vi "Daemon_JETAbout.vi"(6 "Dialog Name":string, 10 "Dialog Parameters":string) -> ()   [LabVIEW 2019]
doc: "JSMA Module Template - Top Level UI 0.2.0.4\nRob Humfeld - Jet Engineering\nCopyright (c) 2019, Jet Engineering"
uses:
  Daemon_JETAbout - Status STYP.ctl
  <userlib>/Jet Labs/JET Panel/JETPanel_Behavior_STYP.ctl
  <userlib>/Jet Engineering/JET_QSM/Code/Private/JET_QSM - Add State [String API].vi
  <vilib>/Utility/error.llb/Trim Whitespace.vi
  <vilib>/Utility/error.llb/Error Cluster From Error Code.vi
  <userlib>/Jet Labs/JET Panel/JETPanel.lvclass
panel:
  in  "exit?":bool
  out "Prompt":string
  out "winSizer 2":string="W"
  out "winSizer 1":string="W"
  out "Recent states before Error (with tick counts) 2":string
  in  "Status":T1
  out "error out":errorcluster
  # "1241 Park Place NE, Ste E, Cedar Rapids, IA 52402\n319.294.6106        http://www.jetinc.net"
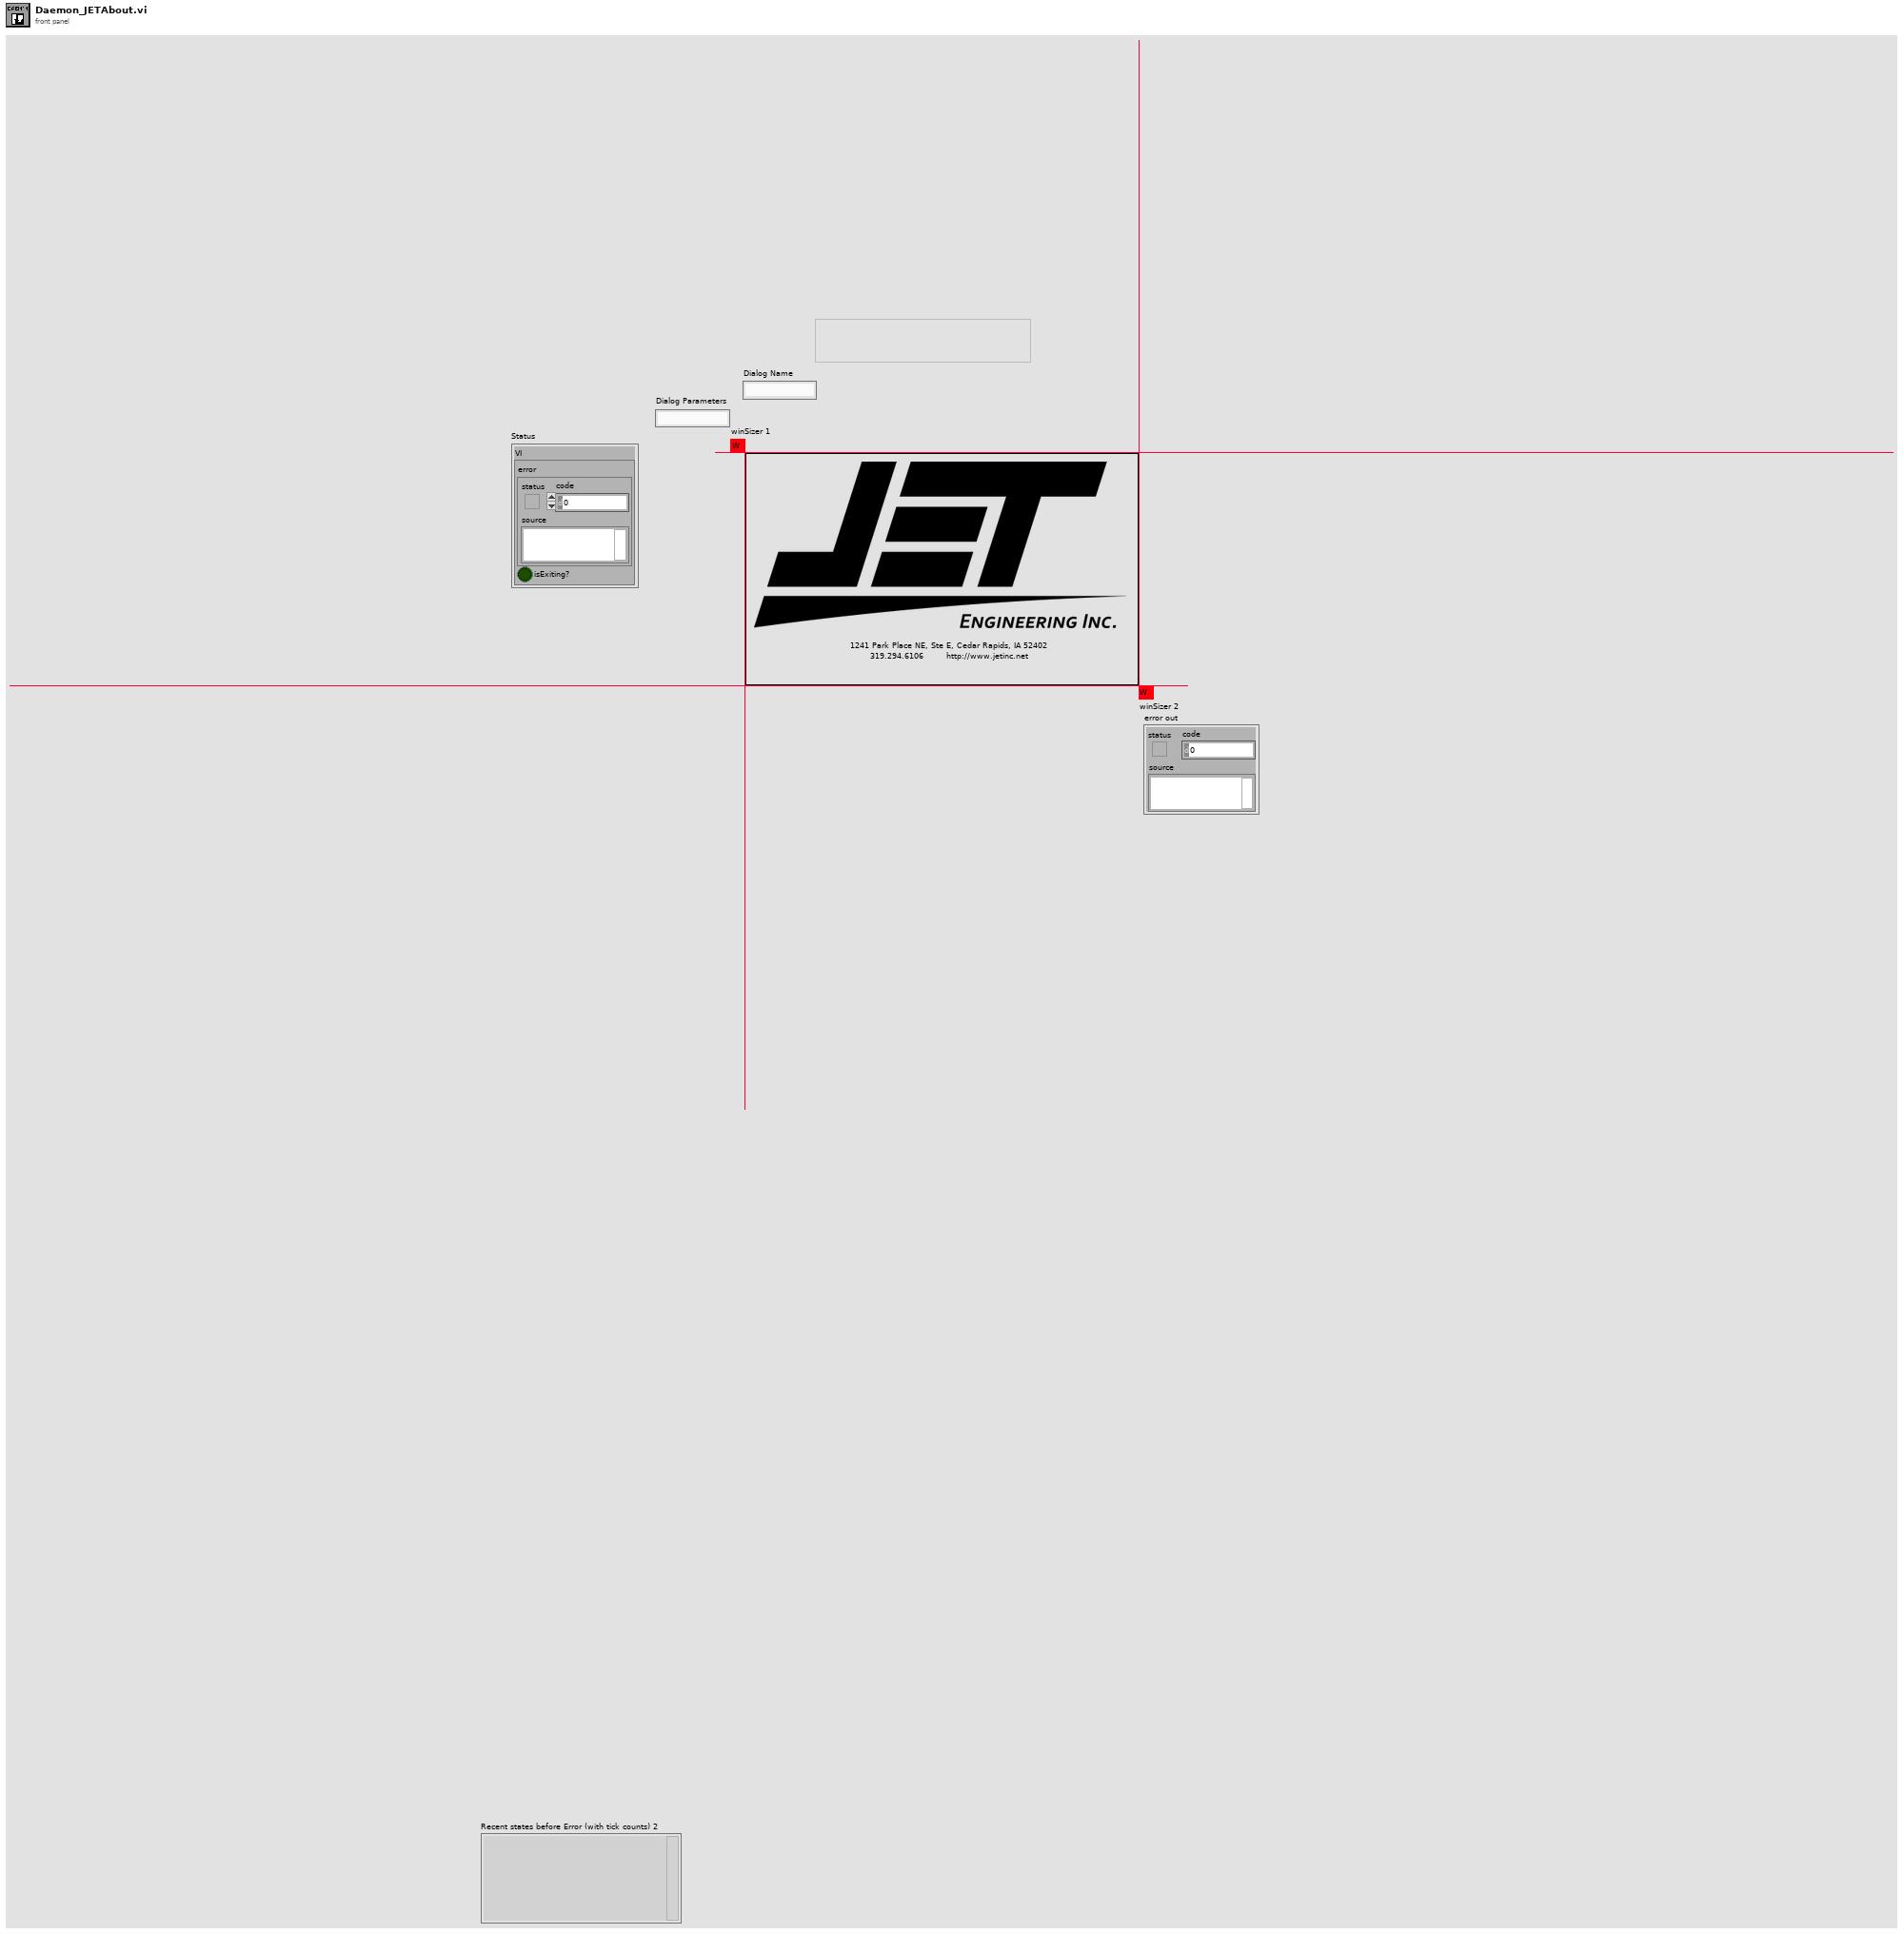
[diagram p1: front panel]
types:
  T1 = typedef "Daemon_JETAbout - Status STYP.ctl" = cluster{"VI":cluster{"error":errorcluster, "isExiting?":bool}}
  T2 = typedef "JETPanel_Behavior_STYP.ctl" = enum32{"Default", "Modal", "Floating", "Floating/Auto-Hide"}
  T3 = typedef "JET_QSM_Refnum STYP.ctl" = cluster{"state":cluster{"queue":refnum<queue>, "idle":string, "error":string, "STOP":string}, "debug":cluster{"enabled?":bool, "queue":refnum<queue>}, "Invalid.option":T4, "QSM.Name":string}
  T4 = typedef "JET_QSM_InvalidOption STYP.ctl" = enum16{"Ignore", "Dialog", "Error"}
  T5 = typedef "JET_QSM_Element STYP.ctl" = cluster{"state":string, "data":variant, "comment":string}
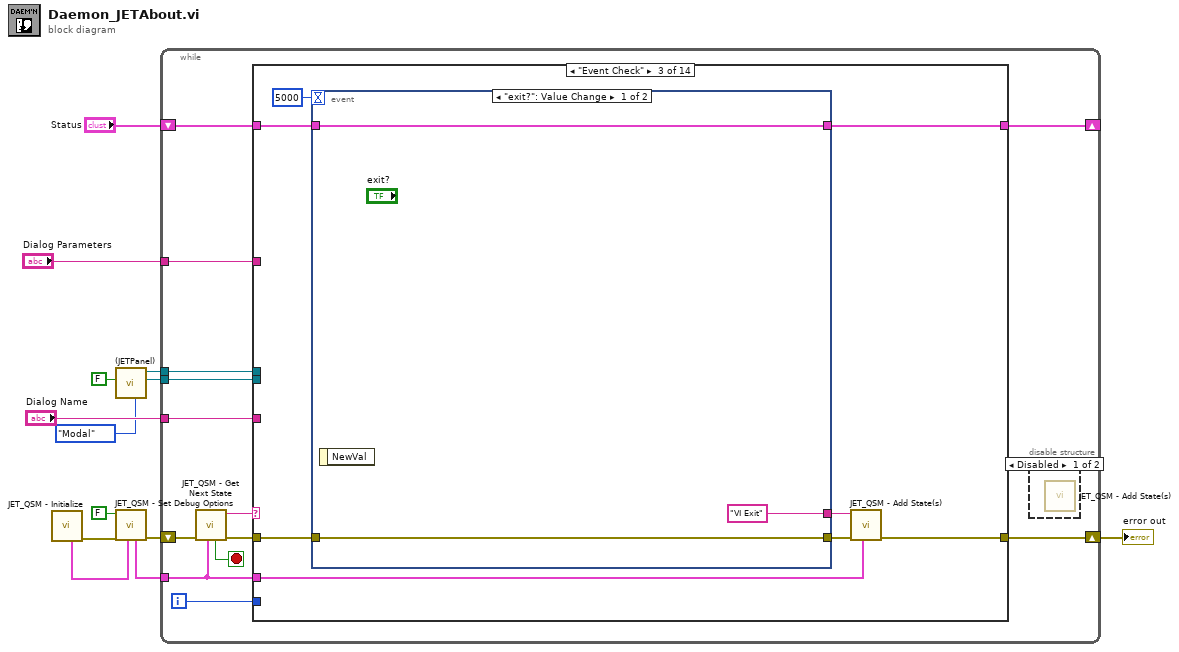
[diagram p0: block diagram]
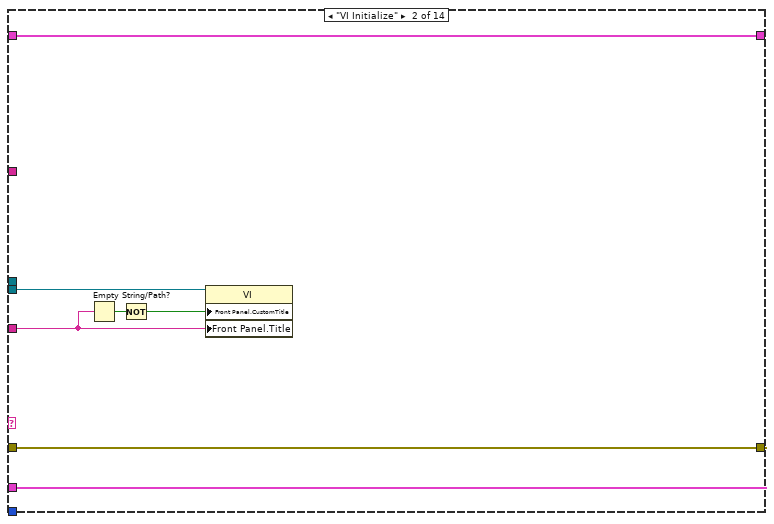
[diagram p4: hidden frame]
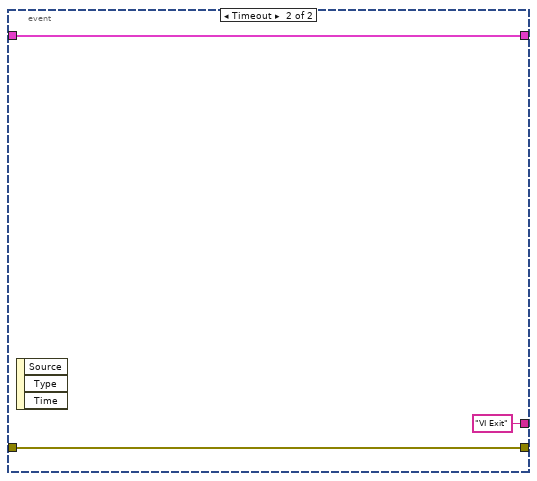
[diagram p5: hidden frame]
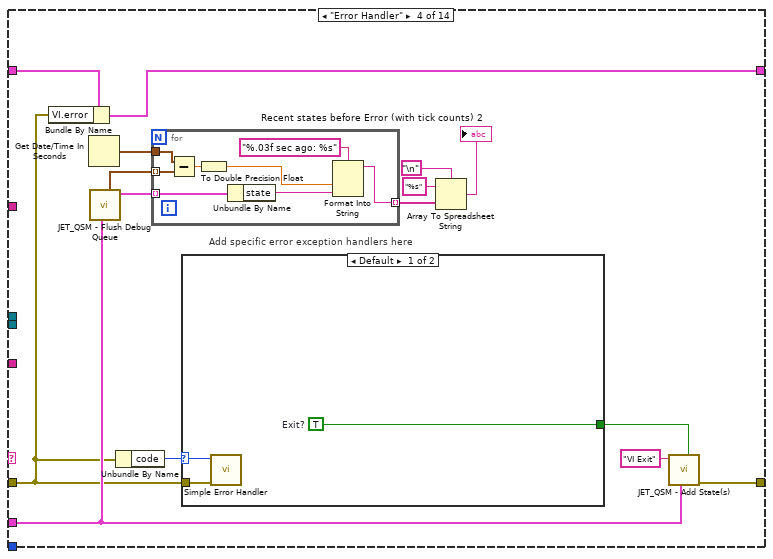
[diagram p6: hidden frame]
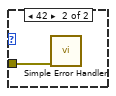
[diagram p7: hidden frame]
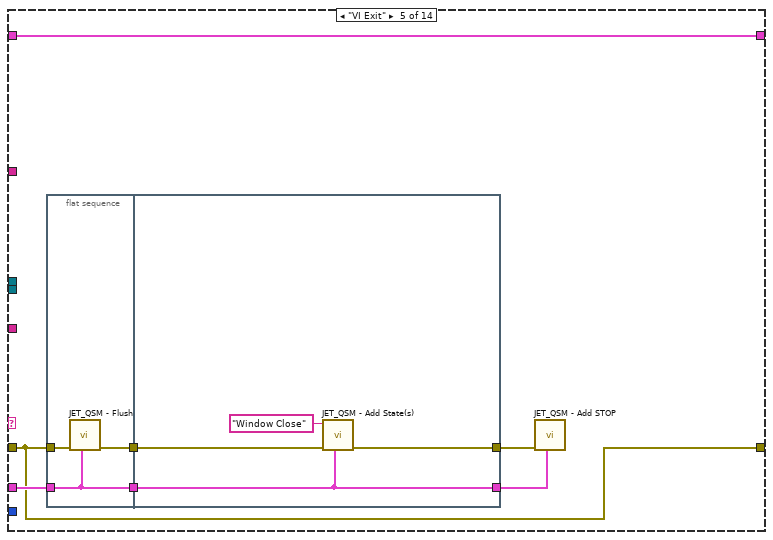
[diagram p8: hidden frame]
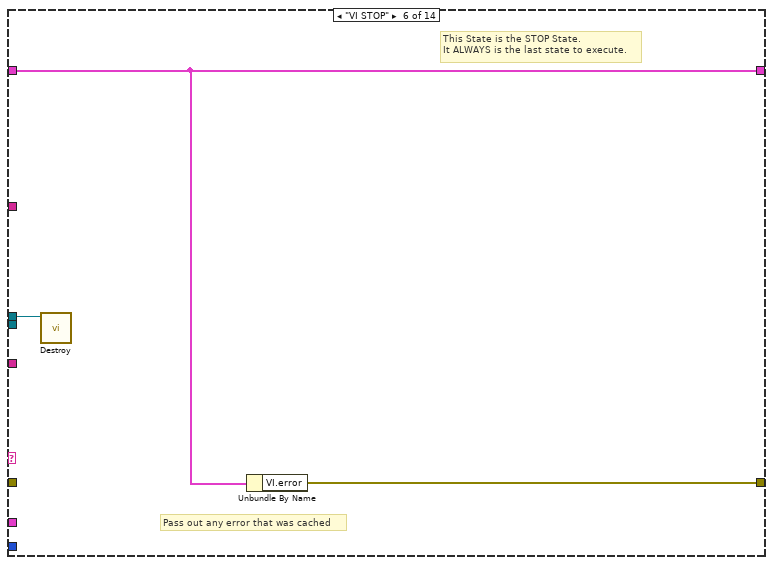
[diagram p9: hidden frame]
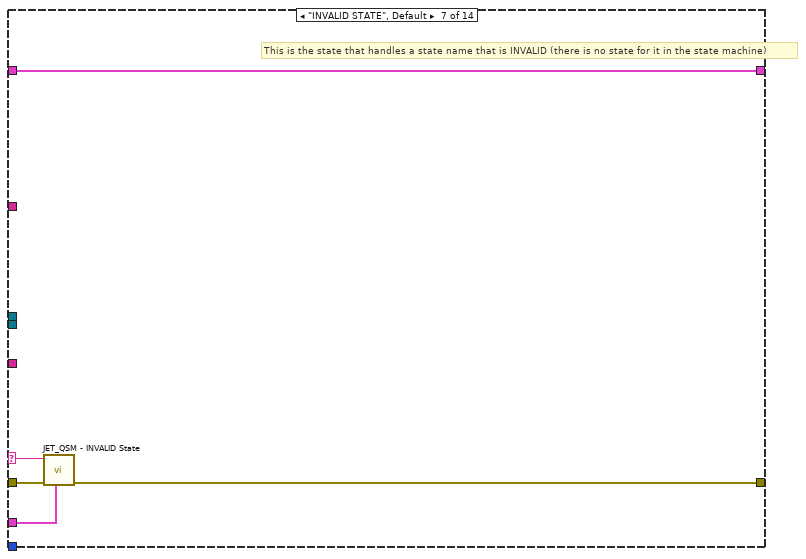
[diagram p10: hidden frame]
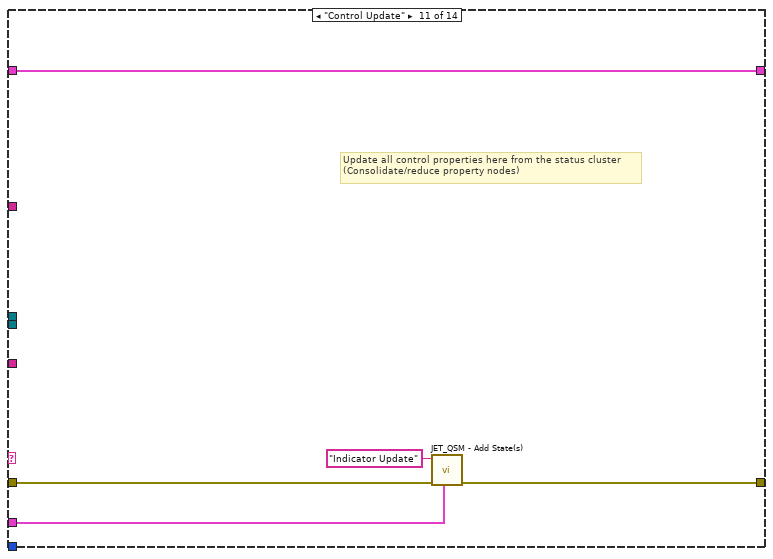
[diagram p14: hidden frame]
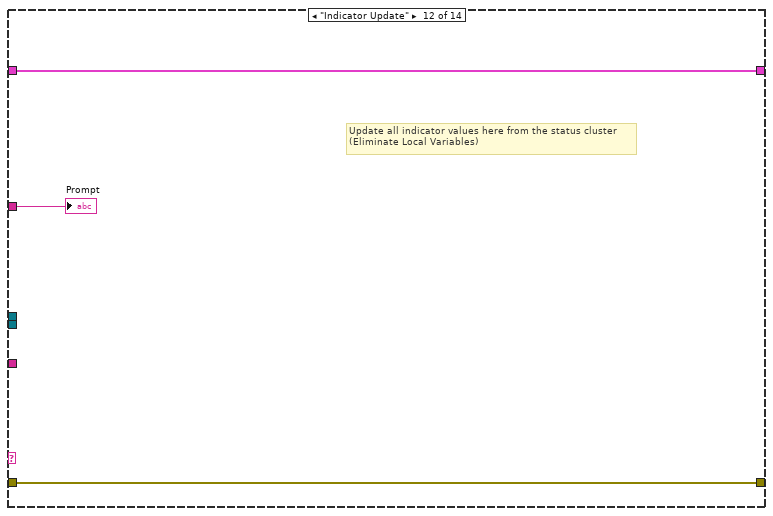
[diagram p15: hidden frame]
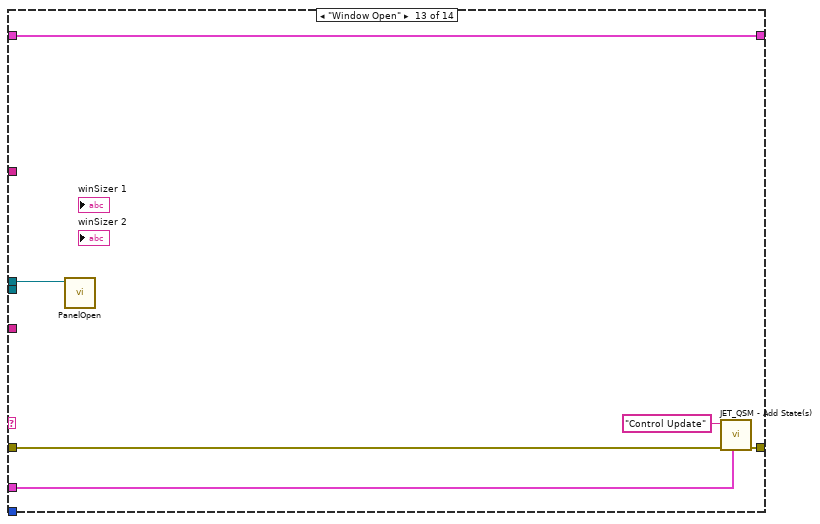
[diagram p16: hidden frame]
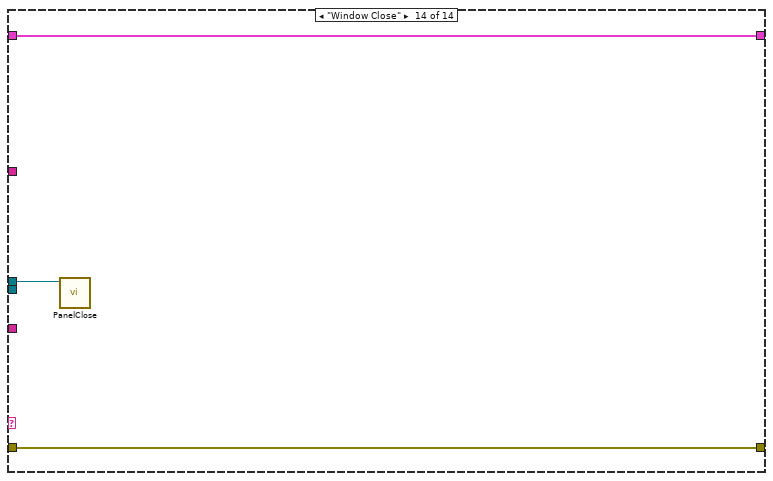
[diagram p17: hidden frame]
diagram:
  n1 = call <userlib>:"JET_QSM - Initialize.vi"() -> ("error out"=w13:errorcluster, "Jet_QSM refnum"=w10:T3)  [unwired: 10 in]
  n2 = call <userlib>:"(JETPanel).vi"("Behavior (Default)"=JETPanel_Behavior_STYP."Modal", "ShowTitleBar? (T)"=FALSE) -> ("VI Refnum"=w4:refnum<vi>, "JETPanel"=w6:refnum<class "JETPanel.lvclass">)  [unwired: 6 in, 2 out]
  n3 = call <userlib>:"JET_QSM - Set Debug Options.vi"("Jet_QSM refnum"=w10, "error in (no error)"=w13, "debug.enabled? (F)"=FALSE) -> ("error out"=w12:errorcluster, "Jet_QSM ref"=w11:T3)  [unwired: 7 in]
  n4 = while {
    tunnel: w11 -> [w22]
    shift-right: [w20] -> _
    shift-left: "Status" -> [w21]
    shift-right: [w19] -> w7
    shift-left: w12 -> [w26]
    tunnel: w6 -> [w17]
    tunnel: "Dialog Parameters" -> [w16]
    tunnel: w4 -> [w15]
    tunnel: "Dialog Name" -> [w14]
    i -> [w18]
    stop <- w23 stop-if-true
    n5 = call <userlib>:"JET_QSM - Get Next State.vi"("Jet_QSM refnum"=w22, "error in (no error)"=w26) -> ("error out"=w25:errorcluster, "state"=w24:string, "Stop Loop?"=w23:bool)  [unwired: 5 in, 2 out]
    n6 = case shown="\"Event Check\"" w24 {
      selector: w24 -> [_ _ _ _ _ _ w98 _ _ _ _ _ _ _]
      tunnel: w25 -> [w27 w37 w42 w54 w79 _ w99 w101 w103 w105 w108 w113 w117 w122]
      tunnel: w22 -> [_ w35 w45 w58 w84 _ w97 _ _ _ w109 _ w118 _]
      tunnel: w21 -> [w28 w29 w44 w53 w82 w94 w100 w102 w104 w106 w111 w114 w120 w123]
      tunnel: [w28 w29 w43 w52 w82 w94 w100 w102 w104 w106 w111 w114 w120 w123] -> w20
      tunnel: [w27 w34 w40 w59 w79 w95 w96 w101 w103 w105 w107 w113 w116 w122] -> w19
      tunnel: w18 -> [_ _ _ _ _ _ _ _ _ _ _ _ _ _]
      tunnel: w17 -> [_ _ _ _ _ w93 _ _ _ _ _ _ w115 w121]
      tunnel: w16 -> [_ _ _ _ _ _ _ _ _ _ _ w112 _ _]
      tunnel: w15 -> [_ w33 _ _ _ _ _ _ _ _ _ _ _ _]
      tunnel: w14 -> [_ w32 _ _ _ _ _ _ _ _ _ _ _ _]
      frame "------ Standard States ------" {
        # "Standard States are required states for a JET_QSM State Machine\n\nTheir names may be changed; use the Initialize function to specify the new names"
        # "This is a section header; the state is never expected to execute"
      }
      frame "VI Initialize" {
        n7 = Empty String/Path?(string/path=w32) -> (empty?=w31:bool)
        n8 = Not(x=w31) -> (.not. x?=w30:bool)
        n9 = property class="VI"(reference=w33, "Front Panel.CustomTitle"=w30, "Front Panel.Title"=w32) -> ()  [unwired: 1 in, 2 out]
        n10 = call-poly <userlib>:"JET_QSM - Add State(s).vi"("Jet_QSM refnum"=w35, "error in (no error)"=w37, "state(s)"="Window Open") -> ("error out"=w34:errorcluster)  [unwired: 8 in]
      }
      frame "Event Check" {
        n11 = event shown="[0] \"exit?\": Value Change" {
          selector: _ -> [_ _]
          dyn-events: _ -> [_ _]
          timeout: 5000 -> [_ _]
          tunnel: w44 -> [w48 w50]
          tunnel: [w48 w50] -> w43
          tunnel: w42 -> [w47 w49]
          tunnel: [w47 w49] -> w41
          tunnel: ["VI Exit" ("state(s)") "VI Exit" ("state(s)")] -> w39
          event "exit?": Value Change {
            n12 = event-data() -> ()  [unwired: 1 in, 1 out]
          }
          event Timeout {
            n13 = event-data() -> ()  [unwired: 1 in, 3 out]
          }
        }
        n14 = call-poly <userlib>:"JET_QSM - Add State(s).vi"("Jet_QSM refnum"=w45, "error in (no error)"=w41, "state(s)"=w39) -> ("error out"=w40:errorcluster)  [unwired: 8 in]
      }
      frame "Error Handler" {
        # "Add specific error exception handlers here"
        n15 = Bundle By Name(cluster=w53, "VI.error"=w54) -> (w52:T1)
        n16 = Get Date/Time In Seconds() -> (seconds since 1Jan1904=w62:timestamp)
        n17 = call <userlib>:"JET_QSM - Flush Debug Queue.vi"("Jet_QSM refnum"=w58) -> ("QSM Elements"=w60:T5[], "Timestamps"=w61:timestamp[])  [unwired: 8 in, 1 out]
        n18 = Unbundle By Name(w54) -> ("code"=w55:i32)
        n19 = for {
          tunnel: w60 -> [w74] mode=indexing
          tunnel: [w72] -> w64 mode=indexing
          tunnel: w62 -> [w69]
          tunnel: w61 -> [w70] mode=indexing
          n20 = Subtract(x=w69, y=w70) -> (x-y=w68:dbl)
          n21 = To Double Precision Float(number=w68) -> (double precision float=w67:dbl)
          n22 = Unbundle By Name(w74) -> ("state"=w73:string)
          n23 = Format Into String(format string="%.03f sec ago: %s", w67, w73) -> (resulting string=w72:string)  [unwired: 2 in, 1 out]
        }
        n24 = case shown="Default" w55 {
          selector: w55 -> [w76 _]
          tunnel: [w77 _] -> w56
          tunnel: w54 -> [w75 w78]
          frame Default {
            w77 = TRUE  # Exit?
            n25 = call <vilib>:"Simple Error Handler.vi"("error code (no error:0)"=w76, "error in (no error)"=w75) -> ()  [unwired: 3 in, 5 out]
          }
          frame 42 {
            n26 = call <vilib>:"Simple Error Handler.vi"("error in (no error)"=w78) -> ()  [unwired: 4 in, 5 out]
          }
        }
        n27 = Array To Spreadsheet String(delimiter (Tab)="\n", array=w64, 3:"%s" ("format string")) -> (spreadsheet string=→"Recent states before Error (with tick counts) 2":string)
        n28 = call-poly <userlib>:"JET_QSM - Add State(s).vi"("act? (T)"=w56, "Jet_QSM refnum"=w58, "state(s)"="VI Exit") -> ("error out"=w59:errorcluster)  [unwired: 8 in]
      }
      frame "VI Exit" {
        n29 = flat-sequence {
          tunnel: w79 -> [w88]
          tunnel: w84 -> [w86]
          tunnel: [w87] -> w81
          tunnel: [w86] -> w80
          tunnel: [w92] -> w83
          tunnel: [w89] -> w85
          tunnel: w81 -> [w90]
          tunnel: w80 -> [w92]
          frame #0 {
            n30 = call <userlib>:"JET_QSM - Flush.vi"("Jet_QSM ref"=w86, "error in (no error)"=w88) -> ("error out"=w87:errorcluster)  [unwired: 8 in, 1 out]
          }
          frame #1 {
            n31 = call-poly <userlib>:"JET_QSM - Add State(s).vi"("Jet_QSM refnum"=w92, "error in (no error)"=w90, "state(s)"="Window Close") -> ("error out"=w89:errorcluster)  [unwired: 8 in]
          }
        }
        n32 = call <userlib>:"JET_QSM - Add STOP.vi"("Jet_QSM refnum"=w83, "error in (no error)"=w85) -> ()  [unwired: 9 in, 1 out]
      }
      frame "VI STOP" {
        # "Pass out any error that was cached"
        # "This State is the STOP State.\nIt ALWAYS is the last state to execute."
        n33 = call-dynamic "Destroy.vi"("JETPanel in"=w93) -> ()  [unwired: 10 in, 1 out]
        n34 = Unbundle By Name(w94) -> ("VI.error"=w95:errorcluster)
      }
      frame "INVALID STATE", Default {
        # "This is the state that handles a state name that is INVALID (there is no state for it in the state machine)"
        n35 = call <userlib>:"JET_QSM - INVALID State.vi"("Jet_QSM refnum"=w97, "error in (no error)"=w99, "state"=w98) -> ("error out"=w96:errorcluster)  [unwired: 8 in]
      }
      frame "------ Menu Commands ------" {
        # "This is a section header; the state is never expected to execute"
      }
      frame "------ Actions  ------" {
        # "This is a section header; the state is never expected to execute"
      }
      frame "------ Window and Panel Control ------" {
        # "This is a section header; the state is never expected to execute"
      }
      frame "Control Update" {
        # "Update all control properties here from the status cluster\n(Consolidate/reduce property nodes)"
        n36 = call-poly <userlib>:"JET_QSM - Add State(s).vi"("Jet_QSM refnum"=w109, "error in (no error)"=w108, "state(s)"="Indicator Update") -> ("error out"=w107:errorcluster)  [unwired: 8 in]
      }
      frame "Indicator Update" {
        # "Update all indicator values here from the status cluster\n(Eliminate Local Variables)"
        "Prompt" <- w112
      }
      frame "Window Open" {
        n37 = call-dynamic "PanelOpen.vi"("JETPanel in"=w115) -> ()  [unwired: 9 in, 2 out]
        n38 = call-poly <userlib>:"JET_QSM - Add State(s).vi"("Jet_QSM refnum"=w118, "error in (no error)"=w117, "state(s)"="Control Update") -> ("error out"=w116:errorcluster)  [unwired: 8 in]
      }
      frame "Window Close" {
        n39 = call-dynamic "PanelClose.vi"("JETPanel"=w121) -> ()  [unwired: 9 in, 2 out]
      }
    }
    n40 = disable-structure shown="Disabled" {
      frame Disabled {
        n41 = call-poly <userlib>:"JET_QSM - Add State(s).vi"() -> ()  [unwired: 11 in, 1 out]
      }
      frame Enabled {
      }
    }
  }
  "error out" <- w7
